vi "Array-Unique Strings.vi"(4 "Strings":string[](array[string])) -> (1 "Unique strings":string[](array[string]))   [LabVIEW 2020]
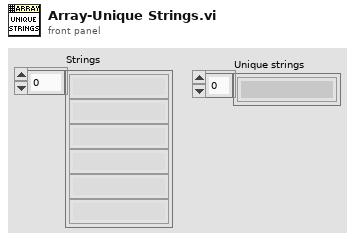
[diagram p1: front panel]
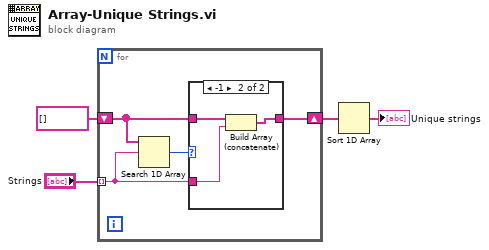
[diagram p0: block diagram]
diagram:
  n1 = for {
    tunnel: "Strings" -> [w6] mode=indexing
    shift-right: [w5] -> w2
    shift-left: string[] [] -> [w7]
    n2 = Search 1D Array(1D array=w7, element=w6) -> (index of element=w8:i32)  [unwired: 1 in]
    n3 = case shown="-1" w8 {
      tunnel: w7 -> [w9 w12]
      tunnel: w6 -> [_ w11]
      tunnel: [w9 w10] -> w5
      frame 0, Default {
      }
      frame -1 {
        n4 = Build Array (concatenate)(w12, w11) -> (w10:string[])
      }
    }
  }
  n5 = Sort 1D Array(array=w2) -> (sorted array=→"Unique strings":string[])
